vi "waitbar.vi"(1 "Number at end of work":u32, 2 "Current Number":u32) -> (0 "Break Computation":bool)   [LabVIEW 2013]
panel:
  in  "stop":bool
  out "Progress":dbl(slide) scale=0.0..1.0
  # "Processing data, please wait."
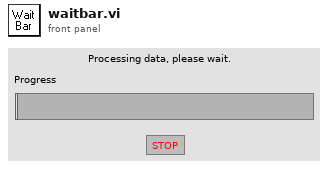
[diagram p1: front panel]
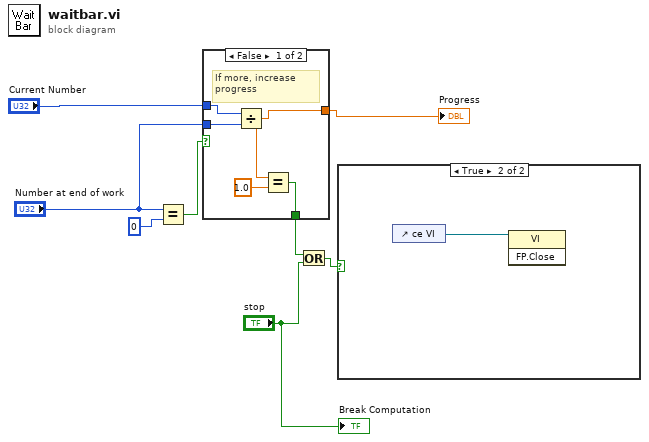
[diagram p0: block diagram]
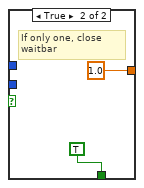
[diagram p2: hidden frame]
diagram:
  n1 = Equal?(x="Number at end of work", y=u32 0) -> (x = y?=w3:bool)
  n2 = case shown="False" w3 {
    tunnel: "Current Number" -> [w13 _]
    tunnel: [w12 1.0] -> w8
    tunnel: [w10 TRUE] -> w7
    tunnel: "Number at end of work" -> [w9 _]
    frame False {
      # "If more, increase progress"
      n3 = Divide(x=w13, y=w9) -> (x/y=w12:dbl)
      n4 = Equal?(x=w12, y=1.0) -> (x = y?=w10:bool)
    }
    frame True {
      # "If only one, close waitbar"
    }
  }
  "Progress" <- w8
  n5 = Or(x=w7, y="stop") -> (x .or. y?=w6:bool)
  n6 = case shown="True" w6 {
    frame False {
    }
    frame True {
      n7 = control-ref of="ce VI"() -> (w16:refnum<vi>)
      n8 = invoke class="VI" method="FP.Close"(reference=w16) -> ()  [unwired: 2 in, 3 out]
    }
  }
  "Break Computation" <- "stop"
